vi "wetter.vi"() -> (3 "Cluster":T1)   [LabVIEW 2018]
panel:
  out "error out":errorcluster
  out "standard error":string
  out "standard output":string
  out "return code":i32
  in  "Super Sayan":bool
  # "Geographical Data"
  # "Geocoder Data"
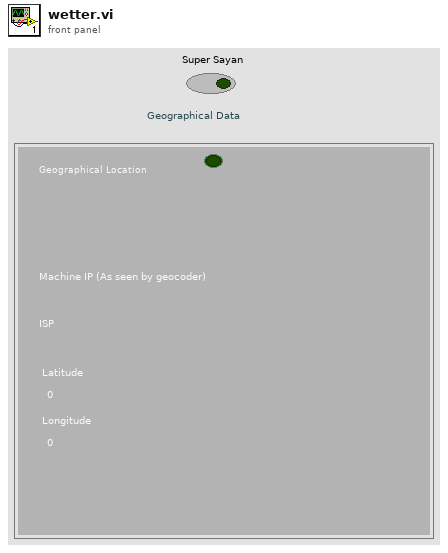
[diagram p1: front panel]
types:
  T1 = cluster{"Geographical Location":string, "Machine IP (As seen by geocoder)":string, "ISP":string, "Latitude":dbl, "Longitude":dbl, "Boolean":bool}
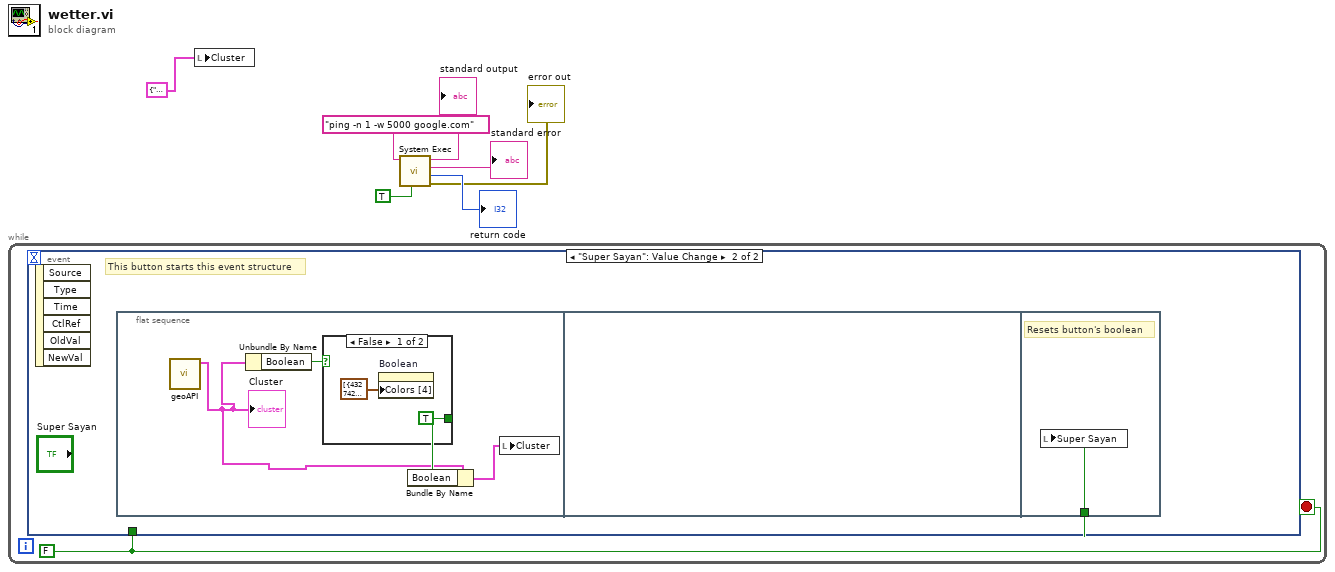
[diagram p0: block diagram]
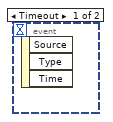
[diagram p2: hidden frame]
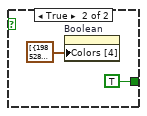
[diagram p3: hidden frame]
diagram:
  n1 = while {
    stop <- w8 stop-if-true
    w8 = FALSE
    n2 = event shown="[1] \"Super Sayan\": Value Change" {
      selector: _ -> [_ _]
      dyn-events: _ -> [_ _]
      timeout: _ -> [_ _]
      tunnel: w8 -> [_ w9]
      event Timeout {
        n3 = event-data() -> ()  [unwired: 1 in, 3 out]
      }
      event "Super Sayan": Value Change {
        # "This button starts this event structure"
        n4 = event-data() -> ()  [unwired: 1 in, 6 out]
        n5 = flat-sequence {
          tunnel: w9 -> [w18]
          frame #0 {
            n6 = call "geoAPI.vi"() -> ("Cluster 2"=w10:T1)  [unwired: 11 in]
            "Cluster" <- w10
            n7 = Unbundle By Name(w10) -> ("Boolean"=w12:bool)
            n8 = case shown="False" w12 {
              tunnel: [TRUE TRUE] -> w13
              frame False {
                n9 = property on="Boolean" class="Bool (strict)"("Colors [4]"=cluster{u32, u32}[] [{4327424, 4327424}, {14431488, 14431488}, {1985280, 1985280}, {6618880, 6618880}]) -> ()  [unwired: 2 in, 2 out]
              }
              frame True {
                n10 = property on="Boolean" class="Bool (strict)"("Colors [4]"=cluster{u32, u32}[] [{1985280, 1985280}, {6618880, 6618880}, {1985280, 1985280}, {6618880, 6618880}]) -> ()  [unwired: 2 in, 2 out]
              }
            }
            n11 = Bundle By Name(cluster=w10, "Boolean"=w13) -> (w11:T1)
            n12 = local write "Cluster"(w11) -> ()
          }
          frame #1 {
          }
          frame #2 {
            # "Resets button's boolean"
            n13 = local write "Super Sayan"(w18) -> ()
          }
        }
      }
    }
  }
  n14 = local write "Cluster"(T1 {"Geographical Location"="", "Machine IP (As seen by geocoder)"="", "ISP"="", "Latitude"=0.0, "Longitude"=0.0, "Boolean"=FALSE} ("Cluster")) -> ()
  n15 = call <vilib>:"System Exec.vi"("run minimized? (F)"=TRUE, "command line"="ping -n 1 -w 5000 google.com") -> ("error out"=→"error out":errorcluster, "return code"=→"return code":i32, "standard error"=→"standard error":string, "standard output"=→"standard output":string)  [unwired: 6 in]
